vi "Pasco Correct Angle.vi"(1 "Given Angle":dbl) -> (0 "Corrected Angle":dbl)   [LabVIEW 2011]
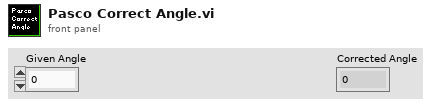
[diagram p1: front panel]
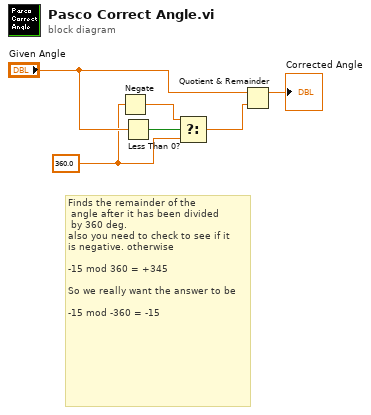
[diagram p0: block diagram]
diagram:
  w1 = 360.0 ("y")
  # "Finds the remainder of the\n angle after it has been divided\n by 360 deg.\nalso you need to check to see if it \nis negative. otherwise\n\n-15 mod 360 = +345\n\nSo we really want the answer to be\n\n-15 mod -360 = -15"
  n1 = Negate(x=w1) -> (-x=w2:dbl)
  n2 = Less Than 0?(x="Given Angle") -> (x < 0?=w4:bool)
  n3 = Select(t=w2, s=w4, f=w1) -> (s? t:f=w5:dbl)
  n4 = Quotient & Remainder(x="Given Angle", y=w5) -> (x-y*floor(x/y)=→"Corrected Angle":dbl)  [unwired: 1 out]
